vi "Get Monitor Total Bounds.vi"(8 "error in (no error)":errorcluster) -> (0 "error out":errorcluster, 3 "window rect":T1)   [LabVIEW 2020, in "MacroAssert.lvlib"]
doc: "This will return an array of clusters with the Horizontal and verticle dimensions in pixels for each display."
uses:
  MacroAssert.lvlib
  System.Windows.Forms
  System.Drawing
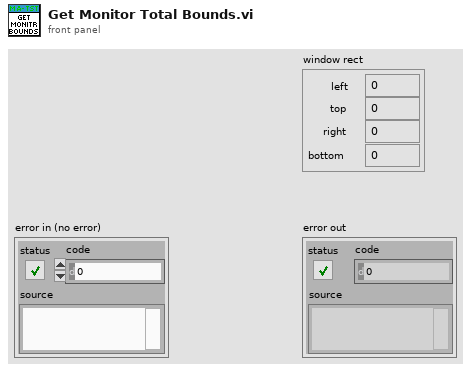
[diagram p1: front panel]
types:
  T1 = cluster{"left":i16, "top":i16, "right":i16, "bottom":i16}
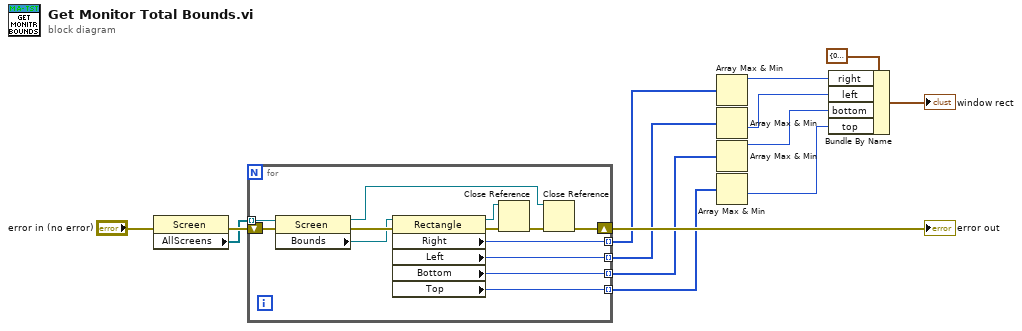
[diagram p0: block diagram]
diagram:
  n1 = property class="Screen"(error in="error in (no error)") -> (error out=w14:errorcluster, "AllScreens"=w12:refnum<k24>[])  [unwired: 1 in, 1 out]
  n2 = for {
    tunnel: w12 -> [w22] mode=indexing
    shift-right: [w20] -> w11
    shift-left: w14 -> [w23]
    tunnel: [w18] -> w10 mode=indexing
    tunnel: [w17] -> w9 mode=indexing
    tunnel: [w16] -> w8 mode=indexing
    tunnel: [w15] -> w7 mode=indexing
    n3 = property class="Screen"(reference=w22, error in=w23) -> (reference out=w26:refnum<k24>, error out=w27:errorcluster, "Bounds"=w19:refnum<k24>)
    n4 = property class="Rectangle"(reference=w19, error in=w27) -> (reference out=w25:refnum<k24>, error out=w24:errorcluster, "Right"=w18:i32, "Left"=w17:i32, "Bottom"=w16:i32, "Top"=w15:i32)
    n5 = Close Reference(reference=w25, error in (no error)=w24) -> (error out=w21:errorcluster)
    n6 = Close Reference(reference=w26, error in (no error)=w21) -> (error out=w20:errorcluster)
  }
  "error out" <- w11
  n7 = Array Max & Min(array=w10) -> (max value=w5:i32)  [unwired: 3 out]
  n8 = Array Max & Min(array=w9) -> (min value=w4:i32)  [unwired: 3 out]
  n9 = Array Max & Min(array=w8) -> (max value=w3:i32)  [unwired: 3 out]
  n10 = Array Max & Min(array=w7) -> (min value=w2:i32)  [unwired: 3 out]
  n11 = Bundle By Name(cluster=T1 {"left"=0, "top"=0, "right"=0, "bottom"=0} ("window rect"), "right"=w5, "left"=w4, "bottom"=w3, "top"=w2) -> (→"window rect":T1)
